vi "Global ingressi analogici.vi"() -> ()   [LabVIEW 2019]
panel:
  in  "Ingressi analogici":dbl[](array[numeric])
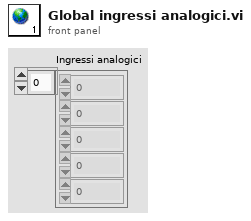
[diagram p1: front panel]
diagram:
